vi "mul_add_24_dc_ht_rnd.vi"(8 "add":fxp<+/-,24,16> format="%#_10g", 10 "Signal":fxp<+/-,24,16>=32.0, 11 "coeff":fxp<+/-,18,2>=0.5) -> (1 "out":fxp<+/-,24,16>)   [LabVIEW 2014]
uses:
  <vilib>/rvi/FXPMathLib/basic elements/DSP48E/simVIs/niFpgaDsp48eSimulationState.ctl
  <vilib>/rvi/FXPMathLib/basic elements/DSP48E/subVIs/niFpgaDsp48eType.ctl
  <vilib>/rvi/FXPMathLib/basic elements/DSP48E/subVIs/niFpgaDsp48eAlumodeOpmodeCarryinselState.ctl
  <vilib>/rvi/FXPMathLib/basic elements/DSP48E/subVIs/niFpgaDsp48eUseMultiplierState.ctl
  <vilib>/rvi/FXPMathLib/basic elements/DSP48E/subVIs/niFpgaDsp48eLogicUnitModeState.ctl
  <vilib>/rvi/FXPMathLib/basic elements/DSP48E/subVIs/niFpgaDsp48eSelectPatternState.ctl
  <vilib>/rvi/FXPMathLib/basic elements/DSP48E/subVIs/niFpgaDsp48eSelectMaskState.ctl
  <vilib>/rvi/FXPMathLib/basic elements/DSP48E/subVIs/niFpgaDsp48eAutoresetState.ctl
  <vilib>/rvi/FXPMathLib/basic elements/DSP48E/simVIs/niFpgaDsp48eResets.ctl
  <vilib>/rvi/FXPMathLib/basic elements/DSP48E/simVIs/niFpgaDsp48eRegisters.ctl
  <vilib>/rvi/FXPMathLib/basic elements/DSP48E/simVIs/niFpgaDsp48eCheckMode.vi
  <vilib>/rvi/FXPMathLib/basic elements/DSP48E/simVIs/niFpgaDsp48eReportInvalidMode.vi
  <vilib>/rvi/FXPMathLib/basic elements/DSP48E/simVIs/niFpgaDsp48eSimBundleEnables.vi
  <vilib>/rvi/FXPMathLib/basic elements/DSP48E/simVIs/niFpgaDsp48eSimMultiplier.vi
  <vilib>/rvi/FXPMathLib/basic elements/DSP48E/simVIs/niFpgaDsp48eSimArithmetic.vi
  <vilib>/rvi/FXPMathLib/basic elements/DSP48E/simVIs/niFpgaDsp48eSimPatternDetect.vi
  <vilib>/rvi/FXPMathLib/basic elements/DSP48E/simVIs/niFpgaDsp48eSimP.vi
  <vilib>/rvi/FXPMathLib/basic elements/DSP48E/simVIs/niFpgaDsp48eSimUpdateState.vi
  <vilib>/rvi/FXPMathLib/basic elements/DSP48E/XNode/niFpgaDsp48e.xnode
panel:
  out "appended array 2":bool[](array[boolean])
  out "appended array":bool[](array[boolean])
  out "number":fxp<+/-,30,16>
  in  "Signal 2":fxp<+/-,24,16>=32.0
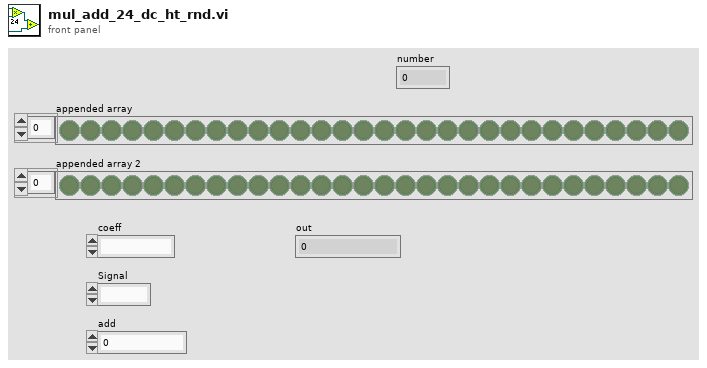
[diagram p1: front panel]
types:
  T1 = cluster{"Boolean array[0]":bool, "Boolean array[1]":bool, "Boolean array[2]":bool, "Boolean array[3]":bool, "Boolean array[4]":bool, "Boolean array[5]":bool, "Boolean array[6]":bool, "Boolean array[7]":bool, "Boolean array[8]":bool, "Boolean array[9]":bool, "Boolean array[10]":bool, "Boolean array[11]":bool, "Boolean array[12]":bool, "Boolean array[13]":bool, "Boolean array[14]":bool, "Boolean array[15]":bool, "Boolean array[16]":bool, "Boolean array[17]":bool, "Boolean array[18]":bool, "Boolean array[19]":bool, "Boolean array[20]":bool, "Boolean array[21]":bool, "Boolean array[22]":bool, "Boolean array[23]":bool}
  T2 = cluster{"Boolean array[0]":bool, "Boolean array[1]":bool, "Boolean array[2]":bool, "Boolean array[3]":bool, "Boolean array[4]":bool, "Boolean array[5]":bool, "Boolean array[6]":bool, "Boolean array[7]":bool, "Boolean array[8]":bool, "Boolean array[9]":bool, "Boolean array[10]":bool, "Boolean array[11]":bool, "Boolean array[12]":bool, "Boolean array[13]":bool, "Boolean array[14]":bool, "Boolean array[15]":bool, "Boolean array[16]":bool, "Boolean array[17]":bool}
  T3 = cluster{"Boolean array[0]":bool, "Boolean array[1]":bool, "Boolean array[2]":bool, "Boolean array[3]":bool, "Boolean array[4]":bool, "Boolean array[5]":bool, "Boolean array[6]":bool, "Boolean array[7]":bool, "Boolean array[8]":bool, "Boolean array[9]":bool, "Boolean array[10]":bool, "Boolean array[11]":bool, "Boolean array[12]":bool, "Boolean array[13]":bool, "Boolean array[14]":bool, "Boolean array[15]":bool, "Boolean array[16]":bool, "Boolean array[17]":bool, "Boolean array[18]":bool, "Boolean array[19]":bool, "Boolean array[20]":bool, "Boolean array[21]":bool, "Boolean array[22]":bool, "Boolean array[23]":bool, "Boolean array[24]":bool, "Boolean array[25]":bool, "Boolean array[26]":bool, "Boolean array[27]":bool, "Boolean array[28]":bool, "Boolean array[29]":bool, "Boolean array[30]":bool, "Boolean array[31]":bool, "Boolean array[32]":bool, "Boolean array[33]":bool, "Boolean array[34]":bool, "Boolean array[35]":bool, "Boolean array[36]":bool, "Boolean array[37]":bool, "Boolean array[38]":bool, "Boolean array[39]":bool, "Boolean array[40]":bool, "Boolean array[41]":bool, "Boolean array[42]":bool, "Boolean array[43]":bool, "Boolean array[44]":bool, "Boolean array[45]":bool, "Boolean array[46]":bool, "Boolean array[47]":bool}
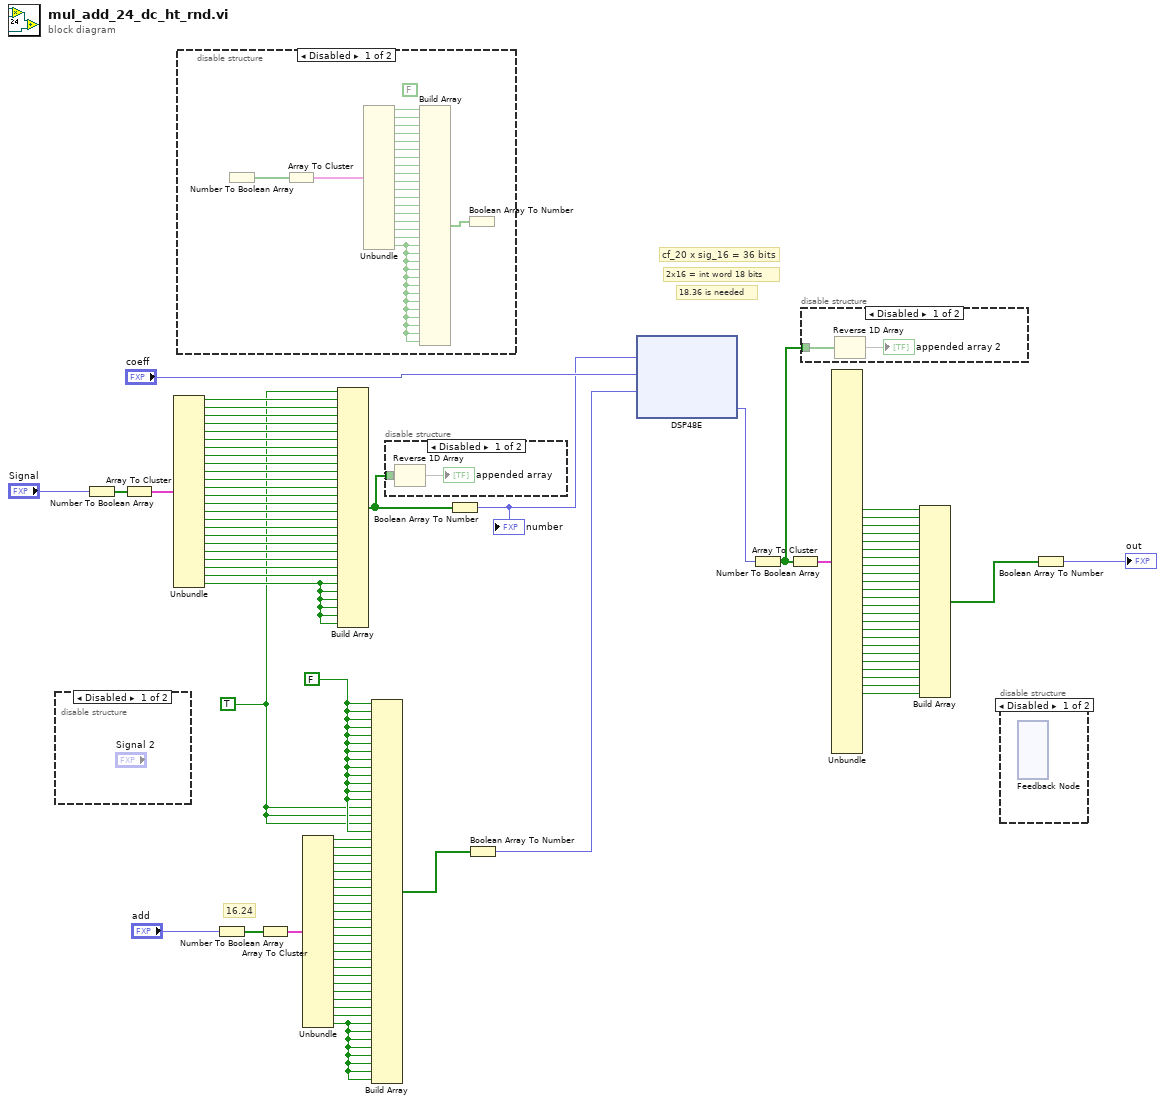
[diagram p0: block diagram]
diagram:
  w1 = TRUE ("Boolean array[0]")
  w2 = FALSE ("Boolean array[0]")
  # "16.24"
  # "18.36 is needed"
  # "2x16 = int word 18 bits"
  # "cf_20 x sig_16 = 36 bits"
  n1 = disable-structure shown="Disabled" {
    frame Disabled {
    }
    frame Enabled {
    }
  }
  n2 = Number To Boolean Array(number="Signal") -> (Boolean array=w26:bool[])
  n3 = Array To Cluster(array=w26) -> (cluster=w90:T1)
  n4 = Unbundle(w90) -> ("Boolean array[0]"=w24:bool, "Boolean array[1]"=w23:bool, "Boolean array[2]"=w22:bool, "Boolean array[3]"=w21:bool, "Boolean array[4]"=w20:bool, "Boolean array[5]"=w19:bool, "Boolean array[6]"=w89:bool, "Boolean array[7]"=w88:bool, "Boolean array[8]"=w87:bool, "Boolean array[9]"=w86:bool, "Boolean array[10]"=w85:bool, "Boolean array[11]"=w84:bool, "Boolean array[12]"=w83:bool, "Boolean array[13]"=w82:bool, "Boolean array[14]"=w81:bool, "Boolean array[15]"=w80:bool, "Boolean array[16]"=w43:bool, "Boolean array[17]"=w42:bool, "Boolean array[18]"=w37:bool, "Boolean array[19]"=w38:bool, "Boolean array[20]"=w39:bool, "Boolean array[21]"=w40:bool, "Boolean array[22]"=w41:bool, "Boolean array[23]"=w12:bool)
  n5 = disable-structure shown="Disabled" {
    frame Disabled {
      (unwired) FALSE ("Boolean array[0]")
      n6 = Number To Boolean Array() -> (Boolean array=w92:bool[])  [unwired: 1 in]
      n7 = Array To Cluster(array=w92) -> (cluster=w94:T2)
      n8 = Unbundle(w94) -> ("Boolean array[0]"=w95:bool, "Boolean array[1]"=w111:bool, "Boolean array[2]"=w96:bool, "Boolean array[3]"=w97:bool, "Boolean array[4]"=w98:bool, "Boolean array[5]"=w99:bool, "Boolean array[6]"=w100:bool, "Boolean array[7]"=w101:bool, "Boolean array[8]"=w102:bool, "Boolean array[9]"=w103:bool, "Boolean array[10]"=w104:bool, "Boolean array[11]"=w105:bool, "Boolean array[12]"=w106:bool, "Boolean array[13]"=w107:bool, "Boolean array[14]"=w108:bool, "Boolean array[15]"=w109:bool, "Boolean array[16]"=w110:bool, "Boolean array[17]"=w91:bool)
      n9 = Build Array(w95, w111, w96, w97, w98, w99, w100, w101, w102, w103, w104, w105, w106, w107, w108, w109, w110, w91, w91, w91, w91, w91, w91, w91, w91, w91, w91, w91, w91, w91) -> (w93:bool[])
      n10 = Boolean Array To Number(Boolean array=w93) -> ()  [unwired: 1 out]
    }
    frame Enabled {
    }
  }
  n11 = Number To Boolean Array(number="add") -> (Boolean array=w79:bool[])
  n12 = Array To Cluster(array=w79) -> (cluster=w78:T1)
  n13 = Unbundle(w78) -> ("Boolean array[0]"=w55:bool, "Boolean array[1]"=w56:bool, "Boolean array[2]"=w57:bool, "Boolean array[3]"=w58:bool, "Boolean array[4]"=w59:bool, "Boolean array[5]"=w60:bool, "Boolean array[6]"=w61:bool, "Boolean array[7]"=w62:bool, "Boolean array[8]"=w63:bool, "Boolean array[9]"=w64:bool, "Boolean array[10]"=w65:bool, "Boolean array[11]"=w66:bool, "Boolean array[12]"=w67:bool, "Boolean array[13]"=w68:bool, "Boolean array[14]"=w69:bool, "Boolean array[15]"=w70:bool, "Boolean array[16]"=w71:bool, "Boolean array[17]"=w72:bool, "Boolean array[18]"=w73:bool, "Boolean array[19]"=w74:bool, "Boolean array[20]"=w75:bool, "Boolean array[21]"=w76:bool, "Boolean array[22]"=w77:bool, "Boolean array[23]"=w3:bool)
  n14 = Build Array(w1, w24, w23, w22, w21, w20, w19, w89, w88, w87, w86, w85, w84, w83, w82, w81, w80, w43, w42, w37, w38, w39, w40, w41, w12, w12, w12, w12, w12, w12) -> (w14:bool[])
  n15 = Build Array(w2, w2, w2, w2, w2, w2, w2, w2, w2, w2, w2, w2, w2, w1, w1, w1, w2, w55, w56, w57, w58, w59, w60, w61, w62, w63, w64, w65, w66, w67, w68, w69, w70, w71, w72, w73, w74, w75, w76, w77, w3, w3, w3, w3, w3, w3, w3, w3) -> (w29:bool[])
  n16 = disable-structure shown="Disabled" {
    disable-tunnel: w14 -> [w113 _]
    frame Disabled {
      n17 = Reverse 1D Array(array=w113) -> (reversed array=→"appended array":bool[])
    }
    frame Enabled {
    }
  }
  n18 = Boolean Array To Number(Boolean array=w14) -> (number=w18:fxp<+/-,30,16>)
  "number" <- w18
  n19 = Boolean Array To Number(Boolean array=w29) -> (number=w4:fxp<+/-,48,18>)
  n20 = xnode ("DSP48E")("a"=w18, "b"="coeff", "c"=w4) -> ("p"=w36:fxp<+/-,48,48>)
  n21 = Number To Boolean Array(number=w36) -> (Boolean array=w13:bool[])
  n22 = Array To Cluster(array=w13) -> (cluster=w54:T3)
  n23 = disable-structure shown="Disabled" {
    disable-tunnel: w13 -> [w114 _]
    frame Disabled {
      n24 = Reverse 1D Array(array=w114) -> (reversed array=→"appended array 2":bool[])
    }
    frame Enabled {
    }
  }
  n25 = Unbundle(w54) -> ("Boolean array[17]"=w11:bool, "Boolean array[18]"=w10:bool, "Boolean array[19]"=w9:bool, "Boolean array[20]"=w8:bool, "Boolean array[21]"=w7:bool, "Boolean array[22]"=w6:bool, "Boolean array[23]"=w5:bool, "Boolean array[24]"=w47:bool, "Boolean array[25]"=w48:bool, "Boolean array[26]"=w49:bool, "Boolean array[27]"=w50:bool, "Boolean array[28]"=w51:bool, "Boolean array[29]"=w52:bool, "Boolean array[30]"=w53:bool, "Boolean array[31]"=w44:bool, "Boolean array[32]"=w45:bool, "Boolean array[33]"=w46:bool, "Boolean array[34]"=w35:bool, "Boolean array[35]"=w34:bool, "Boolean array[36]"=w28:bool, "Boolean array[37]"=w27:bool, "Boolean array[38]"=w16:bool, "Boolean array[39]"=w17:bool, "Boolean array[40]"=w15:bool)  [unwired: 24 out]
  n26 = Build Array(w11, w10, w9, w8, w7, w6, w5, w47, w48, w49, w50, w51, w52, w53, w44, w45, w46, w35, w34, w28, w27, w16, w17, w15) -> (w33:bool[])
  n27 = disable-structure shown="Disabled" {
    frame Disabled {
      n28 = feedback #1() -> ()  [unwired: 2 in]
      n29 = feedback-in #1() -> ()  [unwired: 1 in, 1 out]
    }
    frame Enabled {
    }
  }
  n30 = Boolean Array To Number(Boolean array=w33) -> (number=→"out":fxp<+/-,24,16>)
